vi "PersonnelUIDtoIndex.vi"(8 "error in (no error)":errorcluster, 10 "PUID":string, 11 "Personnel in":refnum<class "Personnel.lvclass">[](array[class])) -> (0 "error out":errorcluster, 1 "Personnel":refnum<class "Personnel.lvclass">, 2 "Index":i32, 3 "Personnel out":refnum<class "Personnel.lvclass">[](array[class]))   [LabVIEW 2015]
uses:
  LVClasses/Personnel/Personnel.lvclass
  LVClasses/Personnel/Personnel.lvclass/Personnel.ctl
  LVClasses/Personnel/Read UniqueID.vi
  <vilib>/Utility/error.llb/Error Cluster From Error Code.vi
  <vilib>/ErrorRing/Error Ring.xnode
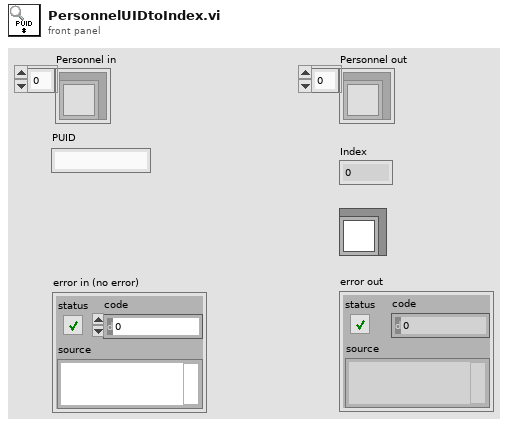
[diagram p1: front panel]
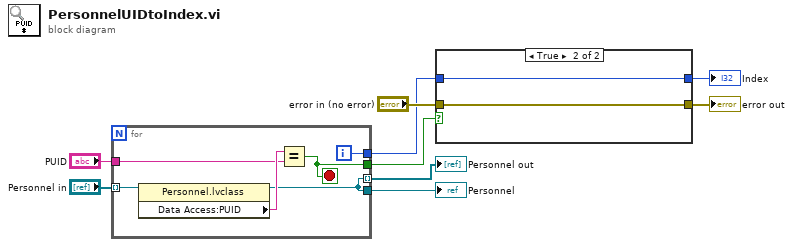
[diagram p0: block diagram]
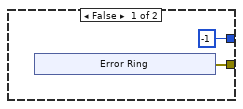
[diagram p2: hidden frame]
diagram:
  n1 = for {
    tunnel: "PUID" -> [w14]
    tunnel: "Personnel in" -> [w13] mode=indexing
    tunnel: [w12] -> w7
    tunnel: [w11] -> w6 mode=indexing
    tunnel: [w11] -> w5
    tunnel: [w10] -> w1
    i -> [w10]
    stop <- w12 stop-if-true
    n2 = property class="Personnel.lvclass"(reference=w13) -> (reference out=w11:refnum<class "Personnel.lvclass">, "Data Access:PUID"=w15:string)  [unwired: 1 in, 1 out]
    n3 = Equal?(x=w15, y=w14) -> (x = y?=w12:bool)
  }
  "Personnel out" <- w6
  "Personnel" <- w5
  n4 = case shown="True" w7 {
    tunnel: "error in (no error)" -> [_ w24]
    tunnel: [w17 w24] -> w3
    tunnel: [-1 ("f") w23] -> w4
    tunnel: w1 -> [_ w23]
    frame False {
      n5 = xnode "Error Ring"() -> ("error out"=w17:errorcluster)
    }
    frame True {
    }
  }
  "error out" <- w3
  "Index" <- w4
